vi "grab data from light matrix.vi"(10 "file path (dialog if empty)":path=path "C:/Users/dhstuart/Box Sync/LT Photometric - 3000 hr Data/LT 01-01.csv", 11 "Color Parameters in":T1) -> (2 "Power Spectral Distribution":cluster{"X":dbl, "Y":dbl}[](graph), 3 "Color Parameters out":T1)   [LabVIEW 2013, in "AvaSpec.lvlib"]
uses:
  AvaSpec.lvlib
  Acquisition/AvaSpec Color Parameters.ctl
  Acquisition/Sphere Indicator.ctl
panel:
  out "Array":dbl[][](array[numeric])
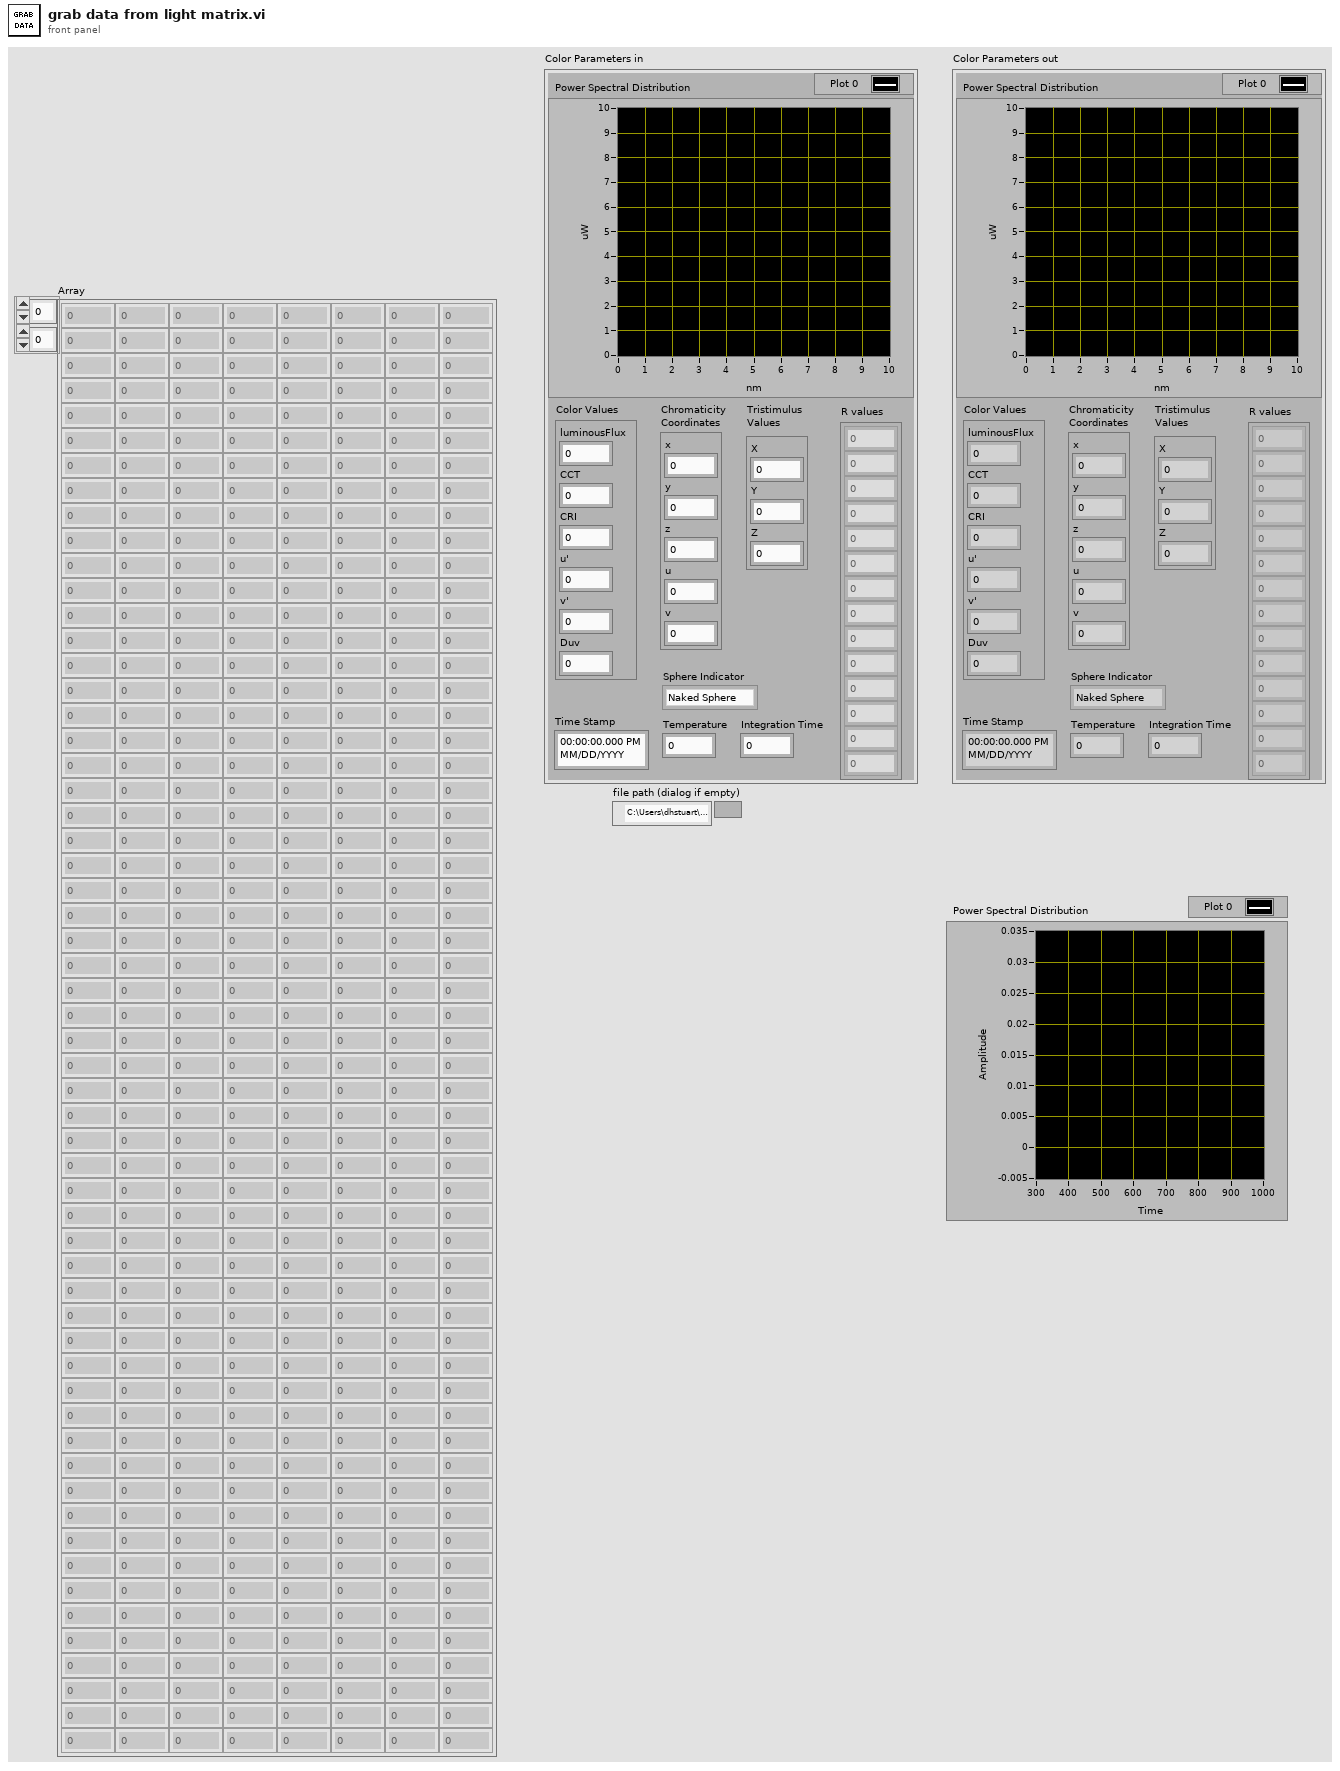
[diagram p1: front panel]
types:
  T1 = typedef "AvaSpec.lvlib/AvaSpec Color Parameters.ctl" = cluster{"Power Spectral Distribution":cluster{"X":dbl, "Y":dbl}[], "Color Values":cluster{"luminousFlux":dbl, "CCT":dbl, "CRI":dbl, "u'":dbl, "v'":dbl, "Duv":dbl}, "R values":dbl[], "Chromaticity \nCoordinates":cluster{"x":dbl, "y":dbl, "z":dbl, "u":dbl, "v":dbl}, "Tristimulus \nValues":cluster{"X":dbl, "Y":dbl, "Z":dbl}, "Time Stamp":timestamp, "Temperature":dbl, "Integration Time":dbl, "Sphere Indicator":T2}
  T2 = typedef "AvaSpec.lvlib/Sphere Indicator.ctl" = enum16{"Naked Sphere", "Insulated Sphere"}
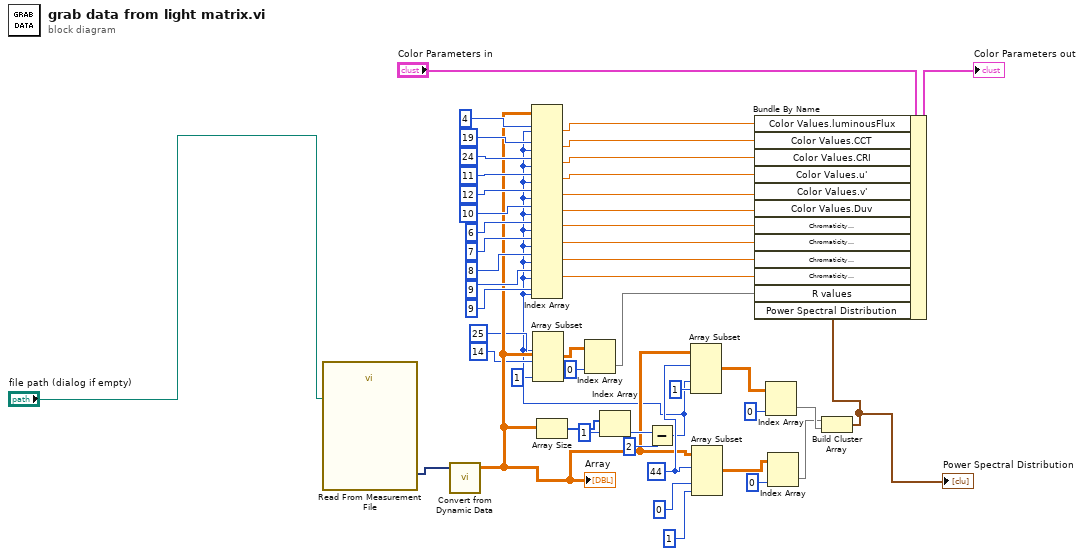
[diagram p0: block diagram]
diagram:
  w41 = 44 ("disabled index (col)")
  n1 = call "Read From Measurement File"("Filename"="file path (dialog if empty)") -> ("Signals"=w47:dynamicdata)  [unwired: 5 in, 5 out]
  n2 = call "Convert from Dynamic Data"("Dynamic Data Type"=w47) -> ("Array"=w16:dbl[][])  [unwired: 3 in]
  "Array" <- w16
  n3 = Array Size(array=w16) -> (size(s)=w46:i32[])
  n4 = Index Array(array=w46, index=1) -> (element=w40:i32)
  n5 = Subtract(x=w40, y=2) -> (x-y=w13:i32)
  n6 = Index Array(array=w16, index (row) #1=4 ("index (row)"), index (col) #1=w13, index (row) #2=19 ("disabled index (row)"), index (col) #2=w13, index (row) #3=24 ("disabled index (row)"), index (col) #3=w13, index (row) #4=11 ("disabled index (row)"), index (col) #4=w13, index (row) #5=12 ("disabled index (row)"), index (col) #5=w13, index (row) #6=10 ("disabled index (row)"), index (col) #6=w13, index (row) #7=6 ("disabled index (row)"), index (col) #7=w13, index (row) #8=7 ("disabled index (row)"), index (col) #8=w13, index (row) #9=8 ("disabled index (row)"), index (col) #9=w13, index (row) #10=9 ("disabled index (row)"), index (col) #10=w13, index (row) #11=9 ("disabled index (row)"), index (col) #11=w13) -> (element #1=w31:dbl, element #2=w30:dbl, element #3=w29:dbl, element #4=w28:dbl, element #5=w27:dbl, element #6=w26:dbl, element #7=w21:dbl, element #8=w20:dbl, element #9=w19:dbl, element #10=w18:dbl)  [unwired: 1 out]
  n7 = Array Subset(array=w16, index (row)=25 ("index"), length (row)=14 ("length"), index (col)=w13, length (col)=1 ("length")) -> (w11:dbl[][])
  n8 = Index Array(array=w11, index (col)=0 ("disabled index (col)")) -> (element=w10:dbl[])  [unwired: 1 in]
  n9 = Array Subset(array=w16, index (row)=w41, index (col)=w13, length (col)=1 ("length")) -> (w9:dbl[][])  [unwired: 1 in]
  n10 = Array Subset(array=w16, index (row)=w41, index (col)=0 ("index"), length (col)=1 ("length")) -> (w8:dbl[][])  [unwired: 1 in]
  n11 = Index Array(array=w9, index (col)=0 ("disabled index (col)")) -> (element=w6:dbl[])  [unwired: 1 in]
  n12 = Index Array(array=w8, index (col)=0 ("disabled index (col)")) -> (element=w5:dbl[])  [unwired: 1 in]
  n13 = Build Cluster Array(w5, w6) -> (w4:cluster{"element":dbl, "element":dbl}[])
  "Power Spectral Distribution" <- w4
  n14 = Bundle By Name(cluster="Color Parameters in", "Color Values.luminousFlux"=w31, "Color Values.CCT"=w30, "Color Values.CRI"=w29, "Color Values.u'"=w28, "Color Values.v'"=w27, "Color Values.Duv"=w26, "Chromaticity \nCoordinates.x"=w21, "Chromaticity \nCoordinates.y"=w20, "Chromaticity \nCoordinates.u"=w19, "Chromaticity \nCoordinates.v"=w18, "R values"=w10, "Power Spectral Distribution"=w4) -> (→"Color Parameters out":T1)
